vi "Overlay.vi"(8 "error in (no error)":errorcluster, 10 "Image In":T1, 11 "Overlay Base in":refnum<class "Analyze Results Distanz.lvclass">) -> (0 "error out":errorcluster, 2 "Image out":T1, 3 "Overlay Base out":refnum<class "Analyze Results Distanz.lvclass">)   [LabVIEW 2020, in "Analyze Results Distanz.lvclass"]
uses:
  Analyze Results Distanz.lvclass
  C:/POLARIS Programme/POLARIS-AS-3-Cams/Submodules/HIJ Vision/Analyze/Results and Overlays/Results Base/Analyze Results Base.lvclass
  <vilib>/vision/Image Controls.llb/IMAQ Image.ctl
  Results Base/Analyze Results Base.lvclass/Analyze Results Base.ctl
  Analyze Results Distanz.lvclass/Analyze Results Distanz.ctl
  Results Base/Read Overlay_.vi
  Results Base/Read Overlay colors.vi
  Results Base/Read Font, Size & Style.vi
  Results Base/Analyze Results Base.lvclass
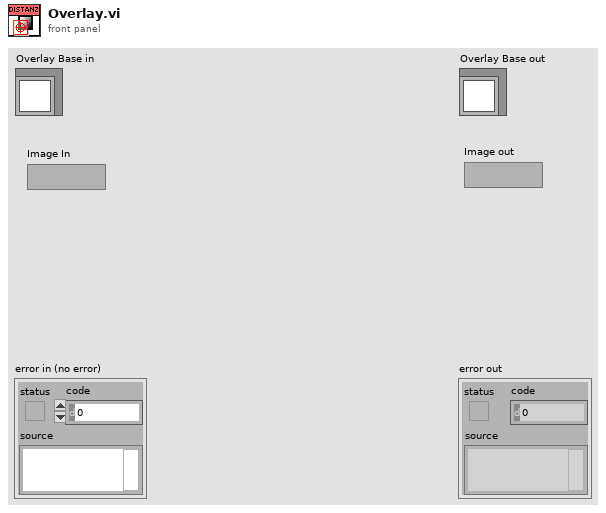
[diagram p1: front panel]
types:
  T1 = typedef "IMAQ Image.ctl" = refnum<image>
  T2 = cluster{"Desired Font (Application)":enum16{"User-specified Font", "Application Font", "System Font", "Dialog Font"}, "[User-specified Font]":cluster{"Font Name":string, "Size":i16, "Strikeout?":bool, "Italic?":bool, "Underline?":bool, "Outline?":bool, "Shadow?":bool, "Bold?":bool, "Rotation Angle":dbl}, "Horizontal Alignment":i16, "Vertical Alignment":i16}
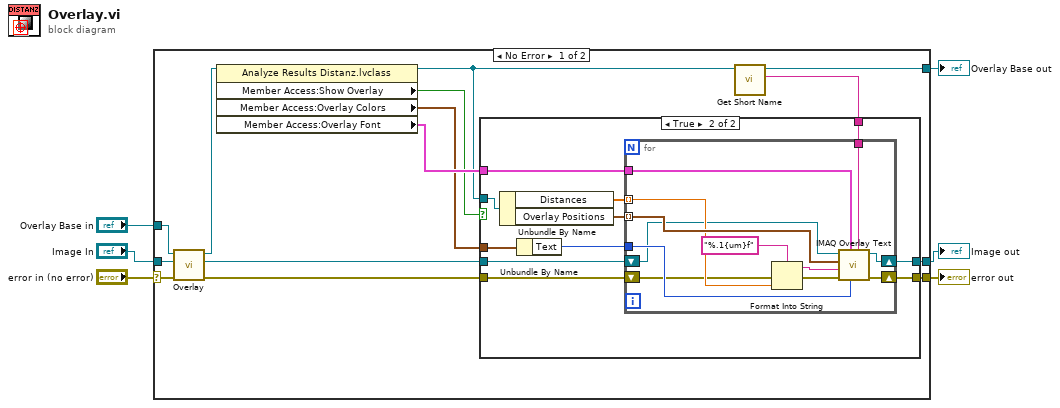
[diagram p0: block diagram]
diagram:
  n1 = case shown="No Error" "error in (no error)" {
    selector: "error in (no error)" -> [w10 w46]
    tunnel: "Image In" -> [w20 w47]
    tunnel: "Overlay Base in" -> [w19 w48]
    tunnel: [w9 w48] -> w4
    tunnel: [w13 w47] -> w3
    tunnel: [w11 w46] -> w2
    frame No Error {
      n2 = call-parent "Overlay.vi"("error in (no error)"=w10, "Image In"=w20, "Overlay Base in"=w19) -> ("error out"=w12:errorcluster, "Image out"=w14:T1, "Overlay Base out"=w18:refnum<class "Analyze Results Distanz.lvclass">)  [unwired: 6 in]
      n3 = property class="Analyze Results Distanz.lvclass"(reference=w18) -> (reference out=w7:refnum<class "Analyze Results Distanz.lvclass">, "Member Access:Show Overlay"=w15:bool, "Member Access:Overlay Colors"=w16:cluster{"Border":u32, "Text":u32}, "Member Access:Overlay Font"=w17:T2)  [unwired: 1 in, 1 out]
      n4 = call-dynamic "Get Short Name.vi"("Analyze Results Base in"=w7) -> ("Short Name"=w8:string, "Analyze Results Base out"=w9:refnum<class "Analyze Results Distanz.lvclass">)  [unwired: 8 in, 1 out]
      n5 = case shown="True" w15 {
        tunnel: w7 -> [_ w33]
        tunnel: w17 -> [_ w32]
        tunnel: w16 -> [_ w29]
        tunnel: w14 -> [w22 w27]
        tunnel: [w22 w26] -> w13
        tunnel: w12 -> [w21 w25]
        tunnel: [w21 w24] -> w11
        tunnel: w8 -> [_ w23]
        frame False {
        }
        frame True {
          n6 = Unbundle By Name(w33) -> ("Distances"=w30:dbl[unit][], "Overlay Positions"=w31:cluster{"x":i16, "y":i16}[])
          n7 = Unbundle By Name(w29) -> ("Text"=w28:u32)
          n8 = for {
            tunnel: w32 -> [w45]
            tunnel: w31 -> [w44] mode=indexing
            tunnel: w30 -> [w43] mode=indexing
            tunnel: w28 -> [w40]
            shift-right: [w38] -> w26
            shift-left: w27 -> [w39]
            shift-right: [w37] -> w24
            shift-left: w25 -> [w36]
            tunnel: w23 -> [w34]
            n9 = Format Into String(format string="%.1{um}f", error in=w36, w43) -> (resulting string=w42:string, error out=w35:errorcluster)  [unwired: 1 in]
            n10 = call "IMAQ Overlay Text"("Group"=w34, "Text Color (black)"=w40, "Font, Size & Style"=w45, "error in (no error)"=w35, "String"=w42, "Origin"=w44, "Image"=w39) -> ("error out"=w37:errorcluster, "Image Out"=w38:T1)  [unwired: 3 in]
          }
        }
      }
    }
    frame Error {
    }
  }
  "error out" <- w2
  "Overlay Base out" <- w4
  "Image out" <- w3
